vi "HVC9 User Main.vi"() -> ()   [LabVIEW 2019, in "HVC9 User.lvlib"]
uses:
  HVC9 User.lvlib
  Servers/HVC9/HVC9 Class/typeDefs/Server State Data.ctl
  Types/HVC9.ctl
  Types/HVC9 gRPC IDs.ctl
  Types/HVC9 Data.ctl
  Servers/HVC9/HVC9 Class/HVC9.lvclass/HVC9.ctl
  Servers/HVC9/HVC9 Class/HVC9.lvclass
panel:
  in  "Stop":bool
  in  "Server Address":string="0.0.0.0:50051"
  in  "Server Certificate File (.crt)":path
  in  "Server Key File (.key)":path
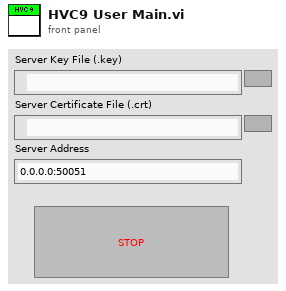
[diagram p1: front panel]
types:
  T1 = typedef "HVC9 User.lvlib/HVC9.ctl" = cluster{"gRPC IDs":T2, "HVC9 Data":T3}
  T2 = typedef "HVC9 User.lvlib/HVC9 gRPC IDs.ctl" = cluster{"Invoke ":u32, "Query":u32, "Register":u32, "OpenNI2564ASession":u32, "CloseNI2564AChannel ":u32, "OpenNI2564AChannel":u32, "DisconnectAllNI2564AChannels":u32, "CloseNI2564ASession":u32, "ResetNI2564A":u32, "OpenNI2564BSession":u32, "CloseNI2564BChannel ":u32, "OpenNI2564BChannel":u32, "DisconnectAllNI2564BChannels":u32, "CloseNI2564BSession":u32, "ResetNI2564B":u32}
  T3 = typedef "HVC9 User.lvlib/HVC9 Data.ctl" = cluster{"NI2564AName":string, "NI2564ASession":refnum<k15>, "NI2564BName":string, "NI2564BSession":refnum<k15>}
  T4 = typedef "HVC9.lvlib/HVC9.lvclass/Server State Data.ctl" = cluster{"Data":string}
  T5 = typedef "HVC9.lvlib/HVC9.lvclass/Server gRPC UEs.ctl" = cluster{"Invoke gRPC UE":refnum<user-event>, "Query gRPC UE":refnum<user-event>, "Register gRPC UE":refnum<user-event>, "OpenNI2564ASession gRPC UE":refnum<user-event>, "CloseNI2564AChannel gRPC UE":refnum<user-event>, "OpenNI2564AChannel gRPC UE":refnum<user-event>, "DisconnectAllNI2564AChannels gRPC UE":refnum<user-event>, "CloseNI2564ASession gRPC UE":refnum<user-event>, "ResetNI2564A gRPC UE":refnum<user-event>, "OpenNI2564BSession gRPC UE":refnum<user-event>, "CloseNI2564BChannel gRPC UE":refnum<user-event>, "OpenNI2564BChannel gRPC UE":refnum<user-event>, "DisconnectAllNI2564BChannels gRPC UE":refnum<user-event>, "CloseNI2564BSession gRPC UE":refnum<user-event>, "ResetNI2564B gRPC UE":refnum<user-event>}
  T6 = typedef "HVC9.lvlib/gprc-lvsupport.lvlib/grpcId.ctl" = u64
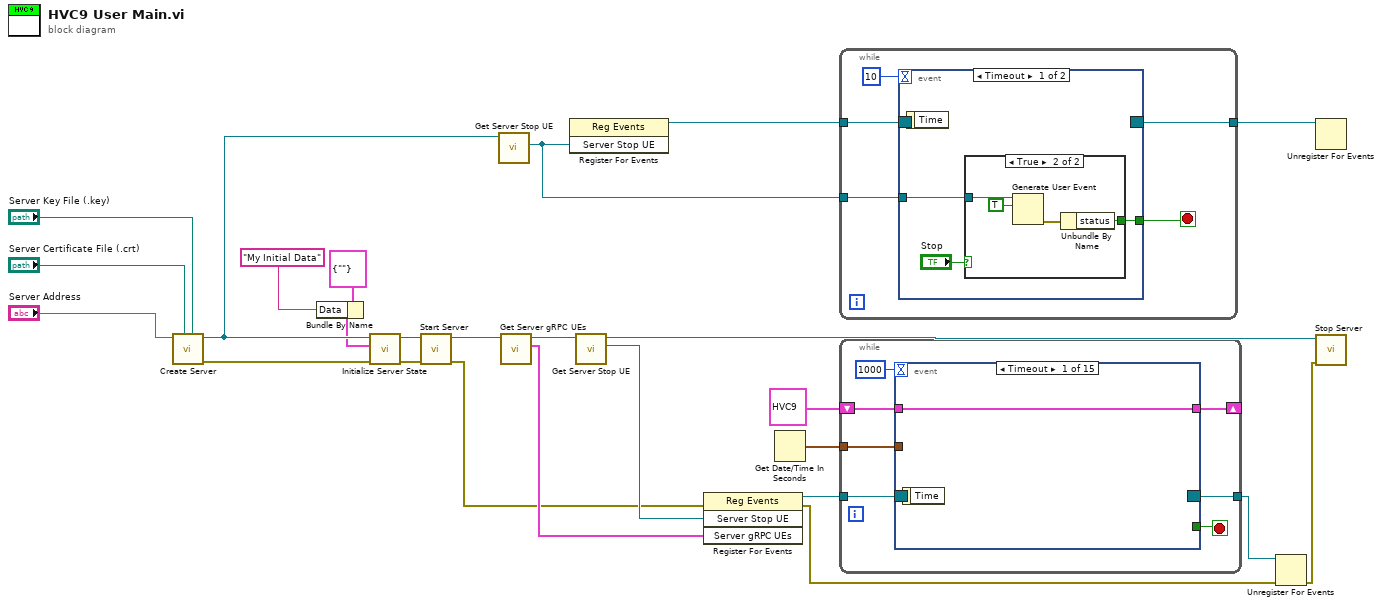
[diagram p0: block diagram]
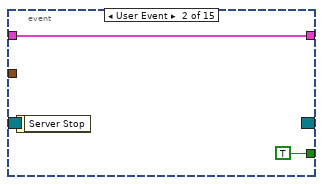
[diagram p2: hidden frame]
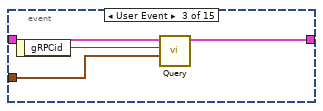
[diagram p3: hidden frame]
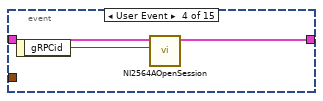
[diagram p4: hidden frame]
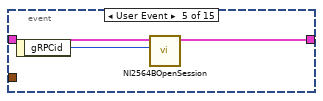
[diagram p5: hidden frame]
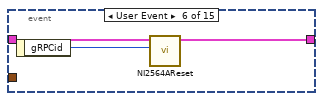
[diagram p6: hidden frame]
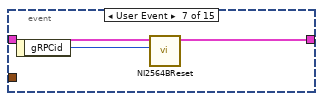
[diagram p7: hidden frame]
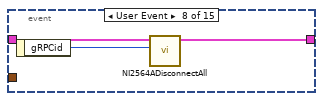
[diagram p8: hidden frame]
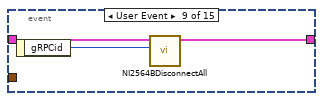
[diagram p9: hidden frame]
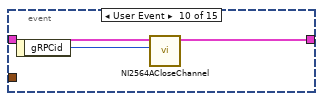
[diagram p10: hidden frame]
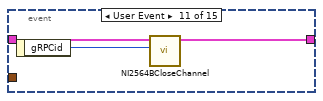
[diagram p11: hidden frame]
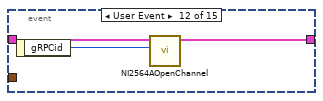
[diagram p12: hidden frame]
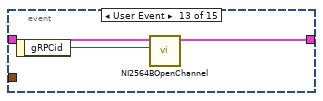
[diagram p13: hidden frame]
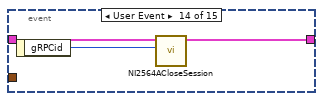
[diagram p14: hidden frame]
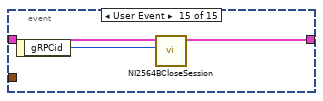
[diagram p15: hidden frame]
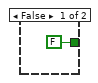
[diagram p16: hidden frame]
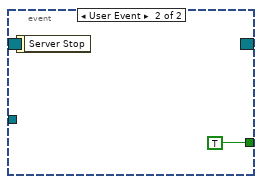
[diagram p17: hidden frame]
diagram:
  n1 = call "Create Server.vi"("Server Key File (.key)"="Server Key File (.key)", "Server Certificate File (.crt)"="Server Certificate File (.crt)", "Server Address"="Server Address") -> ("error out"=w19:errorcluster, "gRPC Server out"=w16:refnum<class "HVC9.lvclass">)  [unwired: 7 in]
  n2 = Bundle By Name(cluster=T4 {"Data"=""} ("Initial State"), "Data"="My Initial Data") -> (w14:T4)
  n3 = call "Initialize Server State.vi"("error in (no error)"=w19, "Initial State"=w14, "gRPC Server in"=w16) -> ("error out"=w18:errorcluster, "gRPC Server out"=w17:refnum<class "HVC9.lvclass">)  [unwired: 7 in]
  n4 = call "Start Server.vi"("error in (no error)"=w18, "gRPC Server in"=w17) -> ("error out"=w2:errorcluster, "gRPC Server out"=w12:refnum<class "HVC9.lvclass">)  [unwired: 8 in]
  n5 = call "Get Server Stop UE.vi"("OOP Server in"=w16) -> ("Server Stop UE"=w20:refnum<user-event>)  [unwired: 9 in, 1 out]
  n6 = call "Get Server gRPC UEs.vi"("OOP Server in"=w12) -> ("Server gRPC UEs"=w7:T5, "OOP Server out"=w9:refnum<class "HVC9.lvclass">)  [unwired: 9 in]
  n7 = register-events(w20) -> (reference out=w22:refnum<event-registration>)  [unwired: 2 in, 1 out]
  n8 = call "Get Server Stop UE.vi"("OOP Server in"=w9) -> ("Server Stop UE"=w8:refnum<user-event>, "OOP Server out"=w11:refnum<class "HVC9.lvclass">)  [unwired: 9 in]
  n9 = register-events(error in=w2, w8, w7) -> (reference out=w6:refnum<event-registration>, error out=w1:errorcluster)  [unwired: 1 in]
  n10 = Get Date/Time In Seconds() -> (seconds since 1Jan1904=w3:timestamp)
  n11 = while {
    tunnel: w20 -> [w30]
    tunnel: w22 -> [w29]
    tunnel: [w27] -> w21
    stop <- w28 stop-if-true
    n12 = event shown="[0] Timeout" {
      selector: w29 -> [_ _]
      dyn-events: [_ _] -> w27
      timeout: 10 -> [_ _]
      tunnel: w30 -> [w33 _]
      tunnel: [w32 TRUE] -> w28
      event Timeout {
        n13 = event-data() -> ()  [unwired: 1 in, 1 out]
        n14 = case shown="True" "Stop" {
          tunnel: w33 -> [_ w36]
          tunnel: [FALSE ("status") w35] -> w32
          frame False {
          }
          frame True {
            n15 = Generate User Event(user event=w36, event data cluster=TRUE ("event data")) -> (error out=w37:errorcluster)  [unwired: 2 in, 1 out]
            n16 = Unbundle By Name(w37) -> ("status"=w35:bool)
          }
        }
      }
      event User Event {
        n17 = event-data() -> ()  [unwired: 1 in, 1 out]
      }
    }
  }
  n18 = while {
    tunnel: w6 -> [w46]
    tunnel: [w44] -> w5
    shift-right: [w41] -> _
    shift-left: T1 {"gRPC IDs"={"Invoke "=0, "Query"=0, "Register"=0, "OpenNI2564ASession"=0, "CloseNI2564AChannel "=0, "OpenNI2564AChannel"=0, "DisconnectAllNI2564AChannels"=0, "CloseNI2564ASession"=0, "ResetNI2564A"=0, "OpenNI2564BSession"=0, "CloseNI2564BChannel "=0, "OpenNI2564BChannel"=0, "DisconnectAllNI2564BChannels"=0, "CloseNI2564BSession"=0, "ResetNI2564B"=0}, "HVC9 Data"={"NI2564AName"="", "NI2564ASession"="", "NI2564BName"="", "NI2564BSession"=""}} ("HVC9") -> [w42]
    tunnel: w3 -> [w40]
    stop <- w45 stop-if-true
    n19 = event "RPC Methods Event Structure" shown="[0] Timeout" {
      selector: w46 -> [_ _ _ _ _ _ _ _ _ _ _ _ _ _ _]
      dyn-events: [_ _ _ _ _ _ _ _ _ _ _ _ _ _ _] -> w44
      timeout: 1000 -> [_ _ _ _ _ _ _ _ _ _ _ _ _ _ _]
      tunnel: [_ TRUE _ _ _ _ _ _ _ _ _ _ _ _ _] -> w45
      tunnel: w42 -> [w47 w48 w53 w55 w58 w61 w64 w67 w70 w73 w76 w79 w82 w85 w88]
      tunnel: [w47 w48 w50 w54 w57 w60 w63 w66 w69 w72 w75 w78 w81 w84 w87] -> w41
      tunnel: w40 -> [_ _ w51 _ _ _ _ _ _ _ _ _ _ _ _]
      event Timeout {
        n20 = event-data() -> ()  [unwired: 1 in, 1 out]
      }
      event User Event {
        n21 = event-data() -> ()  [unwired: 1 in, 1 out]
      }
      event User Event {
        n22 = event-data() -> ("gRPCid"=w52:T6)  [unwired: 1 in]
        n23 = call "Query.vi"("current time"=w51, "gRPCid"=w52, "HVC9 In"=w53) -> ("HVC9 Out"=w50:T1)  [unwired: 7 in, 1 out]
      }
      event User Event {
        n24 = event-data() -> ("gRPCid"=w56:T6)  [unwired: 1 in]
        n25 = call "NI2564AOpenSession.vi"("gRPCid"=w56, "HVC9 In"=w55) -> ("HVC9 Out"=w54:T1)  [unwired: 8 in, 1 out]
      }
      event User Event {
        n26 = event-data() -> ("gRPCid"=w59:T6)  [unwired: 1 in]
        n27 = call "NI2564BOpenSession.vi"("gRPCid"=w59, "HVC9 In"=w58) -> ("HVC9 Out"=w57:T1)  [unwired: 8 in, 1 out]
      }
      event User Event {
        n28 = event-data() -> ("gRPCid"=w62:T6)  [unwired: 1 in]
        n29 = call "NI2564AReset.vi"("gRPCid"=w62, "HVC9 In"=w61) -> ("HVC9 Out"=w60:T1)  [unwired: 8 in, 1 out]
      }
      event User Event {
        n30 = event-data() -> ("gRPCid"=w65:T6)  [unwired: 1 in]
        n31 = call "NI2564BReset.vi"("gRPCid"=w65, "HVC9 In"=w64) -> ("HVC9 Out"=w63:T1)  [unwired: 8 in, 1 out]
      }
      event User Event {
        n32 = event-data() -> ("gRPCid"=w68:T6)  [unwired: 1 in]
        n33 = call "NI2564ADisconnectAll.vi"("gRPCid"=w68, "HVC9 In"=w67) -> ("HVC9 Out"=w66:T1)  [unwired: 8 in, 1 out]
      }
      event User Event {
        n34 = event-data() -> ("gRPCid"=w71:T6)  [unwired: 1 in]
        n35 = call "NI2564BDisconnectAll.vi"("gRPCid"=w71, "HVC9 In"=w70) -> ("HVC9 Out"=w69:T1)  [unwired: 8 in, 1 out]
      }
      event User Event {
        n36 = event-data() -> ("gRPCid"=w74:T6)  [unwired: 1 in]
        n37 = call "NI2564ACloseChannel.vi"("gRPCid"=w74, "HVC9 In"=w73) -> ("HVC9 Out"=w72:T1)  [unwired: 8 in, 1 out]
      }
      event User Event {
        n38 = event-data() -> ("gRPCid"=w77:T6)  [unwired: 1 in]
        n39 = call "NI2564BCloseChannel.vi"("gRPCid"=w77, "HVC9 In"=w76) -> ("HVC9 Out"=w75:T1)  [unwired: 8 in, 1 out]
      }
      event User Event {
        n40 = event-data() -> ("gRPCid"=w80:T6)  [unwired: 1 in]
        n41 = call "NI2564AOpenChannel.vi"("gRPCid"=w80, "HVC9 In"=w79) -> ("HVC9 Out"=w78:T1)  [unwired: 8 in, 1 out]
      }
      event User Event {
        n42 = event-data() -> ("gRPCid"=w83:T6)  [unwired: 1 in]
        n43 = call "NI2564BOpenChannel.vi"("gRPCid"=w83, "HVC9 In"=w82) -> ("HVC9 Out"=w81:T1)  [unwired: 8 in, 1 out]
      }
      event User Event {
        n44 = event-data() -> ("gRPCid"=w86:T6)  [unwired: 1 in]
        n45 = call "NI2564ACloseSession.vi"("gRPCid"=w86, "HVC9 In"=w85) -> ("HVC9 Out"=w84:T1)  [unwired: 8 in, 1 out]
      }
      event User Event {
        n46 = event-data() -> ("gRPCid"=w89:T6)  [unwired: 1 in]
        n47 = call "NI2564BCloseSession.vi"("gRPCid"=w89, "HVC9 In"=w88) -> ("HVC9 Out"=w87:T1)  [unwired: 8 in, 1 out]
      }
    }
  }
  n48 = Unregister For Events(event registration refnum=w5, error in=w1) -> (error out=w10:errorcluster)
  n49 = Unregister For Events(event registration refnum=w21) -> ()  [unwired: 1 in, 1 out]
  n50 = call "Stop Server.vi"("error in (no error)"=w10, "gRPC Server in"=w11) -> ()  [unwired: 9 in, 1 out]
